vi "UHR-Fleezers Control (host) - 12.5.vi"() -> ()   [LabVIEW 2012] (continued)
            "Threshold stored (nm)" <- w2740
          }
        }
      }
      event "FB Trig Integrate": Value Change {
        n1853 = event-data() -> ()  [unwired: 7 out]
        n1854 = local read "FB Trig Integrate"() -> (w2742:u32)
        n1855 = xnode "Read/Write Control"("FPGA VI Reference In"=w2744, "error in"=w2743, "FB Trig Integrate"=w2742) -> ("error out"=w2741:errorcluster)  [unwired: 1 out]
      }
      event "11": Value Change {
        n1856 = event-data() -> ()  [unwired: 7 out]
        n1857 = local read "11"() -> (w2745:bool)
        n1858 = case shown="True" w2745 {
          frame False {
          }
          frame True {
            n1859 = local read "Messages"() -> (w2747:string)
            n1860 = call "Update messages.vi"("Message to add"="You kicked it up to 11!", "Old message string"=w2747) -> ("New message string"=w2748:string)
            n1861 = call <vilib>:"Beep.vi"() -> ()  [unwired: 12 in]
            n1862 = local write "Messages"(w2748) -> ()
          }
        }
      }
      event "Trap Pos. FB ON": Value Change {
        n1863 = event-data() -> ()  [unwired: 7 out]
        n1864 = xnode "Read/Write Control"("FPGA VI Reference In"=w2751, "error in"=w2750, "Force feedback"="Trap Pos. FB ON") -> ()  [unwired: 2 out]
      }
      event "Remove Action Offset": Value Change {
        n1865 = event-data() -> ()  [unwired: 7 out]
        n1866 = local write "Remove Action Offset"(FALSE ("Remove Action Offset")) -> ()
        n1867 = local read "Trap Pos. FB Mult Factor"() -> (w2756:i64)
        n1868 = local read "Trap Pos FB Action"() -> (w2754:i64)
        n1869 = local read "Trap Pos. FB Offset Factor"() -> (w2752:i64)
        n1870 = Multiply(x=w2756, y=w2754) -> (x*y=w2755:i64)
        n1871 = Add(x=w2755, y=w2752) -> (x+y=w2753:i64)
        n1872 = local write "Trap Pos. FB Offset Factor"(w2753) -> ()
        n1873 = xnode "Read/Write Control"("FPGA VI Reference In"=w2759, "error in"=w2758, "Trap Pos. FB Offset Factor"=w2753) -> ()  [unwired: 2 out]
      }
      event "Remove Unwinding Offset": Value Change {
        n1874 = event-data() -> ()  [unwired: 7 out]
        n1875 = local write "Remove Unwinding Offset"(FALSE ("Remove Action Offset")) -> ()
        n1876 = local read "Trap Pos. FB Mult Factor"() -> (w2771:i64)
        n1877 = local read "Trap Pos FB Action"() -> (w2769:i64)
        n1878 = local read "Trap Pos. FB Offset Factor"() -> (w2768:i64)
        n1879 = Multiply(x=w2771, y=w2769) -> (x*y=w2770:i64)
        n1880 = local read "Trap Pos. FB Mult Factor"() -> (w2767:i64)
        n1881 = Add(x=w2770, y=w2768) -> (x+y=w2761:i64)
        n1882 = Multiply(x=32768, y="factor") -> (x*y=w2764:dbl)
        n1883 = Multiply(x=w2764, y=w2767) -> (x*y=w2766:dbl)
        n1884 = Subtract(x=w2761, y=w2766) -> (x-y=w2765:dbl)
        n1885 = To Quad Integer(1:w2765) -> (0:w2760:i64)
        n1886 = xnode "Read/Write Control"("FPGA VI Reference In"=w2774, "error in"=w2773, "Trap Pos. FB Offset Factor"=w2760) -> ()  [unwired: 2 out]
        n1887 = local write "Trap Pos. FB Offset Factor"(w2760) -> ()
      }
      event "Trap Pos. FB Range", "Trap Pos. FB Gains", "Trap Pos. FB Mult Factor", "Trap Pos. FB Offset Factor", "Trap Pos FB Negate Action", "Trap Pos FB Monitor\nT1 or T2", "Differential FB?", "Negate Diff?": Value Change {
        n1888 = event-data() -> ()  [unwired: 7 out]
        n1889 = Unbundle By Name("Trap Pos. FB Gains") -> ("proportional gain (Kc)"=w2777:fxp<+/-,16,8>, "integral gain (Kc*Ts/Ti)"=w2776:fxp<+/-,16,8>, "derivative gain (Kc*Td/Ts)"=w2775:fxp<+/-,16,8>)
        n1890 = local read "Negate Diff?"() -> (w2782:bool)
        n1891 = Unbundle By Name("Trap Pos. FB Range") -> ("output high"=w2780:fxp<+/-,16,1>, "output low"=w2779:fxp<+/-,16,1>)
        n1892 = xnode "Read/Write Control"("FPGA VI Reference In"=w2790, "error in"=w2789, "FB2 output high"=w2780, "FB2 output low"=w2779, "P2"=w2777, "I2"=w2776, "D2"=w2775, "Trap Pos. FB Mult Factor"="Trap Pos. FB Mult Factor", "Trap Pos. FB Offset Factor"="Trap Pos. FB Offset Factor", "Trap Pos FB Negate Action"="Trap Pos FB Negate Action", "Trap Pos FB Monitor T1 or T2"="Trap Pos FB Monitor\nT1 or T2", "AI1 X Scale"="Trap Pos. AI1 X Pre-scale", "Negate Diff?"=w2782, "Diff FB Measurement?"="Differential FB?") -> ()  [unwired: 2 out]
      }
      event "Trap Pos FB SP", "Trap Pos FB SP 2", "Use SP 2": Value Change {
        n1893 = event-data() -> ()  [unwired: 7 out]
        n1894 = Select(t="Trap Pos FB SP 2", s="Use SP 2", f="Trap Pos FB SP") -> (s? t:f=w2791:fxp<+/-,16,1>)
        n1895 = xnode "Read/Write Control"("FPGA VI Reference In"=w2796, "error in"=w2795, "Trap Pos. FB SP"=w2791) -> ()  [unwired: 2 out]
      }
      event "Offset SP2 from SP1": Value Change {
        n1896 = event-data() -> ()  [unwired: 7 out]
        n1897 = local read "Trap Pos FB SP"() -> (w2799:fxp<+/-,16,1>)
        n1898 = Add(x=w2799, y="SP2 Offset") -> (x+y=w2797:fxp<+/-,16,1>)
        n1899 = property on="Trap Pos FB SP 2" class="DigNum (strict)"("Val(Sgnl)"=w2797) -> ()  [unwired: 2 in, 2 out]
        n1900 = local write "Offset SP2 from SP1"(FALSE ("Offset SP2 from SP1")) -> ()
      }
      event "Set Reading to\nSetpoint": Value Change {
        # "This is the actual PID input signal"
        n1901 = event-data() -> ()  [unwired: 7 out]
        n1902 = local write "Set Reading to\nSetpoint"(FALSE ("Set SP to Reading")) -> ()
        n1903 = xnode "Read/Write Control"("FPGA VI Reference In"=w2805, "error in"=w2804) -> ("FPGA VI Reference Out"=w2803:T20, "error out"=w2802:errorcluster, "Trap Pos FB Int-Norm Signal"=w2801:fxp<+/-,16,1>)
        n1904 = local read "Differential FB?"() -> (w2806:bool)
        n1905 = case shown="False" w2806 {
          tunnel: [w2811 w2818] -> w2808
          tunnel: w2801 -> [w2809 w2818]
          frame False {
            n1906 = local read "Trap Pos FB Monitor\nT1 or T2"() -> (w2814:bool)
            n1907 = local read "Trap X AI1 (DMA)"() -> (w2817:T13)
            n1908 = Unbundle By Name(w2817) -> ("Set 1"=w2816:fxp<+/-,16,1>, "Set 2"=w2815:fxp<+/-,16,1>)
            n1909 = Select(t=w2816, s=w2814, f=w2815) -> (s? t:f=w2813:fxp<+/-,16,1>)
            n1910 = Not(x="Set SP Using...") -> (.not. x?=w2810:bool)
            n1911 = Select(t=w2809, s=w2810, f=w2813) -> (s? t:f=w2811:fxp<+/-,16,1>)
          }
          frame True {
          }
        }
        n1912 = xnode "Read/Write Control"("FPGA VI Reference In"=w2803, "error in"=w2802, "Trap Pos. FB SP"=w2808) -> ()  [unwired: 2 out]
        n1913 = local write "Trap Pos FB SP"(w2808) -> ()
      }
      event "Trap Pos. FB Out Scale 2^n": Value Change {
        n1914 = event-data() -> ()  [unwired: 7 out]
        n1915 = Scale By Power Of 2(n="Trap Pos. FB Out Scale 2^n", x=ext 1.0) -> (x*2^n=w2819:ext)
        n1916 = property on="Trap Pos. FB Mult Factor" class="DigNum (strict)"("Val(Sgnl)"=w2819) -> ()  [unwired: 2 in, 2 out]
      }
      event "Trap Pos FB Int Count": Value Change {
        n1917 = event-data() -> ()  [unwired: 7 out]
        n1918 = xnode "Read/Write Control"("FPGA VI Reference In"=w2824, "error in"=w2823, "Trap Pos FB Int Count"="Trap Pos FB Int Count") -> ()  [unwired: 2 out]
      }
      event "Trap pos": Value Change {
        n1919 = event-data() -> ()  [unwired: 7 out]
        n1920 = case shown="True" "Trap pos" {
          frame False {
            n1921 = property on="Trap Delta Graph" class="WFGraph (strict)"("Visible"=TRUE) -> ()  [unwired: 2 in, 2 out]
            n1922 = property on="Saved trap pos" class="WFGraph (strict)"("Visible"=FALSE) -> ()  [unwired: 2 in, 2 out]
          }
          frame True {
            n1923 = property on="Saved trap pos" class="WFGraph (strict)"("Visible"=TRUE) -> ()  [unwired: 2 in, 2 out]
            n1924 = property on="Trap Delta Graph" class="WFGraph (strict)"("Visible"=FALSE) -> ()  [unwired: 2 in, 2 out]
          }
        }
      }
    }
    "error out 2" <- w1634
    n1925 = node-c288() -> ()  [unwired: 2 out]
  }
  n1926 = while "Duncan's play event loop" {
    stop <- w2831 stop-if-true
    n1927 = Create User Event(user event datatype=TRUE ("Boolean")) -> (user event=w2832:refnum<user-event>)  [unwired: 1 in, 1 out]
    n1928 = Create User Event(user event datatype=TRUE ("Boolean")) -> (user event=w2839:refnum<user-event>)  [unwired: 1 in, 1 out]
    n1929 = global write "Global for fluorescence simulation mean (30 samples), (power series).vi" "Red Signal"(w2832) -> ()
    n1930 = global write "Global for fluorescence simulation mean (30 samples), (power series).vi" "Green Signal"(w2839) -> ()
    n1931 = register-events(w2839, w2832) -> (reference out=w2838:refnum<event-registration>)  [unwired: 2 in, 1 out]
    n1932 = event shown="[1] \"Get Fluorophore\": Value Change" {
      selector: w2838 -> [_ _ _ _]
      dyn-events: _ -> [_ _ _ _]
      timeout: 100 -> [_ _ _ _]
      event Timeout {
        n1933 = event-data() -> ()  [unwired: 1 in, 2 out]
      }
      event "Get Fluorophore": Value Change {
        n1934 = event-data() -> ("OldVal"=w2841:bool)  [unwired: 1 in, 4 out]
        n1935 = case shown="True" w2841 {
          selector: w2841 -> [_ w2842]
          frame False {
          }
          frame True {
            n1936 = property on="Move to Position 3" class="Bool"("Val(Sgnl)"=w2842) -> ()  [unwired: 2 in, 2 out]
            n1937 = case shown="1" "Numeric" {
              frame 0, Default {
              }
              frame 1 {
                n1938 = property on="Green Laser ON" class="Bool (strict)"("Val(Sgnl)"=TRUE ("Value (Signaling)")) -> ()  [unwired: 2 in, 2 out]
              }
              frame 2 {
                n1939 = property on="Red Laser ON" class="Bool (strict)"("Val(Sgnl)"=TRUE) -> ()  [unwired: 2 in, 2 out]
              }
            }
          }
        }
      }
      event User Event {
        n1940 = event-data() -> ("Boolean"=w2846:bool)  [unwired: 1 in, 3 out]
        "Green Fluorophore" <- w2846
        n1941 = property on="Get Fluorophore" class="Bool (strict)"("Val(Sgnl)"=w2846) -> ()  [unwired: 2 in, 2 out]
      }
      event User Event {
        n1942 = event-data() -> ("Boolean"=w2847:bool)  [unwired: 1 in, 3 out]
        "Red Fluorophore" <- w2847
        n1943 = property on="Get Fluorophore" class="Bool (strict)"("Val(Sgnl)"=w2847) -> ()  [unwired: 2 in, 2 out]
      }
    }
    n1944 = property on="Get Fluorophore" class="Bool (strict)"("Val(Sgnl)"="Get Fluorophore") -> ()  [unwired: 2 in, 2 out]
    n1945 = Wait (ms)(milliseconds to wait=u32 100) -> ()  [unwired: 1 out]
    n1946 = local read "Stop All"() -> (w2830:bool)
    n1947 = Or(x=w2830, y="stop") -> (x .or. y?=w2831:bool)
  }
  n1948 = timed-loop "Mouse control: trap position (AOM deflection), set confocal spot from image" {
    tunnel: [w2849] -> w207
    tunnel: w13 -> [w2848]
    timing: w129 -> [_]
    timing-out: [_] -> w128
    stop <- w2849 stop-if-true
    n1949 = node-c288() -> ()  [unwired: 2 out]
    n1950 = event shown="[0] \"Pane\": Mouse Down" {
      selector: _ -> [_ _]
      dyn-events: _ -> [_ _]
      timeout: _ -> [_ _]
      tunnel: w2848 -> [w2852 _]
      event Mouse Down {
        n1951 = event-data() -> ("Time"=w2854:u32, "Coords"=w2853:T7, "Button"=w2855:u16)  [unwired: 6 out]
        n1952 = case shown="1" w2855 {
          tunnel: w2854 -> [_ _ w2961]
          tunnel: w2853 -> [_ w2892 w2959]
          tunnel: w2852 -> [_ _ w2957]
          frame 0, Default {
          }
          frame 1 {
            n1953 = property on="APD 2" class="ImageControl"() -> ("Displayed Image Position"=w2862:cluster{"Left":i32, "Top":i32})  [unwired: 2 in, 2 out]
            n1954 = property on="APD 1" class="ImageControl"() -> ("Displayed Image Position"=w2891:cluster{"Left":i32, "Top":i32})  [unwired: 2 in, 2 out]
            n1955 = property on="Detection Laser X" class="ImageControl"() -> ("Displayed Image Position"=w2888:cluster{"Left":i32, "Top":i32})  [unwired: 2 in, 2 out]
            n1956 = property on="Detection Laser Y" class="ImageControl"() -> ("Displayed Image Position"=w2887:cluster{"Left":i32, "Top":i32})  [unwired: 2 in, 2 out]
            n1957 = property on="APD 2" class="ImageControl"() -> ("Displayed Image Size"=w2861:cluster{"Width":u32, "Height":u32})  [unwired: 2 in, 2 out]
            n1958 = property on="APD 1" class="ImageControl"() -> ("Displayed Image Size"=w2889:cluster{"Width":u32, "Height":u32})  [unwired: 2 in, 2 out]
            n1959 = property on="Detection Laser X" class="ImageControl"() -> ("Displayed Image Size"=w2890:cluster{"Width":u32, "Height":u32})  [unwired: 2 in, 2 out]
            n1960 = property on="Detection Laser Y" class="ImageControl"() -> ("Displayed Image Size"=w2886:cluster{"Width":u32, "Height":u32})  [unwired: 2 in, 2 out]
            n1961 = Unbundle By Name(w2861) -> ("Width"=w2858:u32, "Height"=w2857:u32)
            n1962 = Unbundle By Name(w2862) -> ("Left"=w2860:i32, "Top"=w2859:i32)
            n1963 = Unbundle By Name(w2889) -> ("Width"=w2883:u32, "Height"=w2882:u32)
            n1964 = Unbundle By Name(w2890) -> ("Width"=w2879:u32, "Height"=w2878:u32)
            n1965 = Unbundle By Name(w2886) -> ("Width"=w2875:u32, "Height"=w2874:u32)
            n1966 = Unbundle By Name(w2891) -> ("Left"=w2885:i32, "Top"=w2884:i32)
            n1967 = Unbundle By Name(w2888) -> ("Left"=w2881:i32, "Top"=w2880:i32)
            n1968 = Unbundle By Name(w2887) -> ("Left"=w2877:i32, "Top"=w2876:i32)
            n1969 = Bundle("Left"=w2860, "Top"=w2859, "Width"=w2858, "Height"=w2857) -> (w2856:T32)  [unwired: 1 in]
            n1970 = Bundle("Left"=w2885, "Top"=w2884, "Width"=w2883, "Height"=w2882) -> (w2873:T32)  [unwired: 1 in]
            n1971 = Bundle("Left"=w2881, "Top"=w2880, "Width"=w2879, "Height"=w2878) -> (w2872:T32)  [unwired: 1 in]
            n1972 = Bundle("Left"=w2877, "Top"=w2876, "Width"=w2875, "Height"=w2874) -> (w2871:T32)  [unwired: 1 in]
            n1973 = Build Cluster Array(w2856, w2873, w2872, w2871) -> (w2870:T33)
            n1974 = for {
              tunnel: w2892 -> [w2903]
              tunnel: w2870 -> [w2904] mode=indexing
              shift-right: [w2901] -> w2868
              shift-left: TRUE -> [w2902]
              shift-right: [w2900] -> w2866
              shift-left: _ -> [w2896]
              shift-right: [w2899] -> w2865
              shift-left: _ -> [w2895]
              shift-right: [w2898] -> w2864
              shift-left: _ -> [w2894]
              shift-right: [w2897] -> w2863
              shift-left: _ -> [w2893]
              n1975 = case shown="True" w2902 {
                selector: w2902 -> [w2909 _]
                tunnel: w2904 -> [_ w2918]
                tunnel: w2903 -> [_ w2916]
                tunnel: [w2909 w2914] -> w2901
                tunnel: [w2908 w2913] -> w2900
                tunnel: [w2907 w2912] -> w2899
                tunnel: [w2906 w2911] -> w2898
                tunnel: [w2905 w2910] -> w2897
                tunnel: w2896 -> [w2908 _]
                tunnel: w2895 -> [w2907 _]
                tunnel: w2894 -> [w2906 _]
                tunnel: w2893 -> [w2905 _]
                frame False {
                }
                frame True {
                  n1976 = Unbundle(w2918) -> (w2917:T32)
                  n1977 = call "isclickinwindow.vi"("Image Param"=w2917, "Point32"=w2916) -> ("4 Y"=w2910:i32, "3 Height"=w2911:i32, "2 X"=w2912:i32, "1 Width"=w2913:i32, "In image?"=w2915:bool)  [unwired: 1 in]
                  n1978 = Not(x=w2915) -> (.not. x?=w2914:bool)
                }
              }
            }
            n1979 = Not(x=w2868) -> (.not. x?=w2867:bool)
            n1980 = case shown="True" w2867 {
              tunnel: w2865 -> [_ w2932]
              tunnel: w2863 -> [_ w2931]
              tunnel: w2866 -> [_ w2930]
              tunnel: w2864 -> [_ w2929]
              frame False {
              }
              frame True {
                w2919 = FALSE ("Get Point")
                n1981 = local read "Scan lines (y)"() -> (w2934:u64)
                n1982 = disable-structure shown="Disabled" {
                  frame Disabled {
                  }
                  frame Enabled {
                  }
                }
                n1983 = local read "Actual MCL Inc (V)"() -> (w2928:dbl)
                n1984 = local read "Scan steps (MCL)"() -> (w2933:u64)
                n1985 = Divide "Y Pix/step"(x=w2929, y=w2934) -> (x/y=w2941:dbl)
                n1986 = Divide "Y V/pix"(x=w2928, y=w2941) -> (x/y=w2940:dbl)
                n1987 = Divide "Y half step offset"(x=w2928, y=2.0) -> (x/y=w2942:dbl)
                n1988 = Divide "X pix/step"(x=w2930, y=w2933) -> (x/y=w2939:dbl)
                n1989 = Negate(x=w2942) -> (-x=w2943:dbl)
                n1990 = local read "Initial Y"() -> (w2949:dbl)
                n1991 = Multiply(x=w2931, y=w2940) -> (x*y=w2950:dbl)
                n1992 = Divide "X half step offset"(x=w2928, y=2.0) -> (x/y=w2936:dbl)
                n1993 = Divide "X V/pix"(x=w2928, y=w2939) -> (x/y=w2938:dbl)
                n1994 = Multiply(x=w2928, y=w2933) -> (x*y=w2945:dbl)
                n1995 = Compound Arithmetic op=ADD(w2943, w2950, w2949) -> (w2920:dbl)
                "Pointer Y (V)" <- w2920
                n1996 = Multiply(x=w2938, y=w2932) -> (x*y=w2947:dbl)
                n1997 = Negate(x=w2936) -> (-x=w2935:dbl)
                n1998 = local read "Initial X"() -> (w2948:dbl)
                n1999 = Negate(x=w2947) -> (-x=w2946:dbl)
                n2000 = Compound Arithmetic op=ADD(w2935, w2945, w2948, w2946) -> (w2921:dbl)
                "Pointer X (V)" <- w2921
                n2001 = case shown="True" "Set High F Confocal Spot (X-Y)" {
                  tunnel: w2921 -> [_ w2951]
                  tunnel: w2920 -> [_ w2952]
                  frame False {
                  }
                  frame True {
                    "Confocal Y 2 (V)" <- w2952
                    "Confocal X 2 (V)" <- w2951
                  }
                }
                n2002 = Or(x="Set X Only", y="Set Confocal Spot (X-Y)") -> (x .or. y?=w2924:bool)
                n2003 = Or(x="Set Confocal Spot (X-Y)", y="Set Y Only") -> (x .or. y?=w2923:bool)
                n2004 = case shown="True" w2924 {
                  tunnel: w2921 -> [_ w2953]
                  frame False {
                  }
                  frame True {
                    n2005 = property on="AO2" class="Slide (strict)"("Val(Sgnl)"=w2953) -> ()  [unwired: 2 in, 2 out]
                    "Confocal X 1 (V)" <- w2953
                  }
                }
                n2006 = case shown="True" w2923 {
                  tunnel: w2920 -> [_ w2954]
                  frame False {
                  }
                  frame True {
                    n2007 = property on="AO1" class="Slide (strict)"("Val(Sgnl)"=w2954) -> ()  [unwired: 2 in, 2 out]
                    "Confocal Y 1 (V)" <- w2954
                  }
                }
                n2008 = local write "Set High F Confocal Spot (X-Y)"(w2919) -> ()
                n2009 = local write "Set Confocal Spot (X-Y)"(w2919) -> ()
                n2010 = local write "Set X Only"(w2919) -> ()
                n2011 = local write "Set Y Only"(w2919) -> ()
              }
            }
          }
          frame 3 {
            n2012 = local read "BD 2 Frequency 1 (MHz)"() -> (w2955:dbl)
            n2013 = local read "BD 1 Frequency 1 (MHz)"() -> (w2956:dbl)
            n2014 = local write "Manipulating Trap"(TRUE ("Manipulating Trap")) -> ()
            n2015 = local write "Coords"(T7 {"Horizontal"=0, "Vertical"=0} ("Coords")) -> ()
            n2016 = while {
              tunnel: w2961 -> [w2966]
              tunnel: w2959 -> [w2965]
              tunnel: w2957 -> [w2964]
              tunnel: w2956 -> [w2963]
              tunnel: w2955 -> [w2962]
              stop <- w2967 stop-if-true
              n2017 = event shown="[0] \"Pane\": Mouse Move" {
                selector: _ -> [_ _]
                dyn-events: _ -> [_ _]
                timeout: _ -> [_ _]
                tunnel: ["Force Manip Abort" w3031] -> w2967
                tunnel: w2966 -> [w2974 _]
                tunnel: w2965 -> [w2972 _]
                tunnel: w2964 -> [w2971 _]
                tunnel: w2963 -> [w2970 _]
                tunnel: w2962 -> [w2969 _]
                event Mouse Move {
                  n2018 = event-data() -> ("Time"=w2975:u32, "Coords"=w2976:T7)  [unwired: 3 out]
                  n2019 = Less?(x=w2975, y=w2974) -> (x < y?=w2973:bool)
                  n2020 = case "Makes sure old motion events prior to mouse click aren't used" shown="False" w2973 {
                    tunnel: w2976 -> [w3018 _]
                    tunnel: w2972 -> [w3019 _]
                    tunnel: w2971 -> [w2996 _]
                    tunnel: w2970 -> [w2992 _]
                    tunnel: w2969 -> [w2991 _]
                    frame False {
                      n2021 = Subtract(x=w3018, y=w3019) -> (x-y=w3017:T7)
                      "Coords" <- w3017
                      n2022 = local read "Y RF Frequency Limits (MHz)"() -> (w2977:T16)
                      n2023 = To Double Precision Float(number=w3017) -> (double precision float=w3016:cluster{"Horizontal":dbl, "Vertical":dbl})
                      n2024 = Multiply(x=cluster{"Horizontal":dbl, "Vertical":dbl} {"Horizontal"=-1.0, "Vertical"=1.0}, y="Manipulation Scaling") -> (x*y=w3012:cluster{"Horizontal":dbl, "Vertical":dbl})
                      n2025 = local read "X RF Frequency Limits (MHz)"() -> (w2978:T16)
                      n2026 = Multiply(x=w3016, y=w3012) -> (x*y=w3014:cluster{"Horizontal":dbl, "Vertical":dbl})
                      n2027 = Unbundle By Name(w3014) -> ("Horizontal"=w3009:dbl, "Vertical"=w3013:dbl)
                      n2028 = Unbundle By Name(w2977) -> ("Maximum"=w2980:dbl, "Minimum"=w2979:dbl)
                      n2029 = Boolean To (0,1)(Boolean="Manip. X?") -> (0, 1=w3007:i16)
                      n2030 = Boolean To (0,1)(Boolean="Manip. Y?") -> (0, 1=w3004:i16)
                      n2031 = local read "BD 1 Frequency 2 (MHz)"() -> (w2994:dbl)
                      n2032 = Multiply(x=w3013, y=w3004) -> (x*y=w3006:dbl)
                      n2033 = Multiply(x=w3007, y=w3009) -> (x*y=w3010:dbl)
                      n2034 = local read "BD 2 Frequency 2 (MHz)"() -> (w2993:dbl)
                      n2035 = Unbundle By Name(w2978) -> ("Maximum"=w2982:dbl, "Minimum"=w2981:dbl)
                      n2036 = Add(x=w2991, y=w3006) -> (x+y=w2984:dbl)
                      n2037 = Add(x=w2992, y=w3010) -> (x+y=w2986:dbl)
                      n2038 = In Range and Coerce(upper limit=w2982, x=w2986, lower limit=w2981) -> (coerced(x)=w2985:dbl)  [unwired: 1 out]
                      n2039 = In Range and Coerce(upper limit=w2980, x=w2984, lower limit=w2979) -> (coerced(x)=w2983:dbl)  [unwired: 1 out]
                      n2040 = Subtract(x=w2985, y=w2994) -> (x-y=w3003:dbl)
                      n2041 = Subtract(x=w2983, y=w2993) -> (x-y=w3002:dbl)
                      n2042 = Square(x=w3003) -> (x^2=w3001:dbl)
                      n2043 = Square(x=w3002) -> (x^2=w3000:dbl)
                      n2044 = Add(x=w3001, y=w3000) -> (x+y=w2999:dbl)
                      n2045 = Square Root(x=w2999) -> (sqrt(x)=w2995:dbl)
                      n2046 = In Range and Coerce(upper limit="Limit Max (MHz)", x=w2995, lower limit="Limit Min (MHz)") -> (In Range?=w2988:bool)  [unwired: 1 out]
                      n2047 = Not(x="Limits Enable") -> (.not. x?=w2987:bool)
                      n2048 = Or(x=w2988, y=w2987) -> (x .or. y?=w2989:bool)
                      n2049 = case shown="True" w2989 {
                        tunnel: w2996 -> [_ w3029]
                        tunnel: w2995 -> [_ w3020]
                        tunnel: w2985 -> [_ w3027]
                        tunnel: w2994 -> [_ w3026]
                        tunnel: w2983 -> [_ w3025]
                        tunnel: w2993 -> [_ w3024]
                        tunnel: w2978 -> [_ w3022]
                        tunnel: w2977 -> [_ w3021]
                        frame False {
                        }
                        frame True {
                          n2050 = local read "BD 1 Frequency 3 (MHz)"() -> (w3028:dbl)
                          n2051 = local read "BD 2 Frequency 3 (MHz)"() -> (w3023:dbl)
                          n2052 = local write "Trap Delta (MHz)"(w3020) -> ()
                          n2053 = call "set RF board frequency - interlace.vi"("Board 2 Frequency Limits"=w3021, "Board 1 Frequency Limits"=w3022, "FPGA VI Reference In"=w3029, "Board 2 Frequency 3 (MHz)"=w3023, "Board 1 Frequency 3 (MHz)"=w3028, "Board 2 Frequency 2 (MHz)"=w3024, "Board 2 Frequency 1 (MHz)"=w3025, "Board 1 Frequency 2 (MHz)"=w3026, "Board 1 Frequency 1  (MHz)"=w3027) -> ()  [unwired: 1 in, 2 out]
                          n2054 = local write "BD 2 Frequency 1 (MHz)"(w3025) -> ()
                          n2055 = local write "BD 1 Frequency 1 (MHz)"(w3027) -> ()
                        }
                      }
                    }
                    frame True {
                    }
                  }
                }
                event Mouse Up {
                  n2056 = event-data() -> ("Button"=w3030:u16)  [unwired: 8 out]
                  n2057 = case shown="3" w3030 {
                    tunnel: [FALSE TRUE] -> w3031
                    frame 0, Default {
                    }
                    frame 3 {
                      n2058 = local read "Trap Delta (MHz)"() -> (w3033:dbl)
                      n2059 = property on="Initial delta (MHz)" class="DigNum (strict)"("Val(Sgnl)"=w3033) -> ()  [unwired: 2 in, 2 out]
                      n2060 = local write "Manipulating Trap"(FALSE ("Manipulating Trap")) -> ()
                    }
                  }
                }
              }
            }
          }
        }
      }
      event Mouse Move {
        n2061 = event-data() -> ()  [unwired: 6 out]
      }
    }
    n2062 = local read "Stop All"() -> (w2849:bool)
    n2063 = node-c288() -> ()  [unwired: 2 out]
  }
  n2064 = timed-loop "Main data acquisition loop (get data, process data for display, and save data to disk)" {
    tunnel: w12 -> [w3345]
    tunnel: w88 -> [w3344]
    tunnel: [w3374] -> w292
    tunnel: [w3369] -> w290
    timing: w200 -> [_]
    timing-out: [_] -> w199
    tunnel: w105 -> [w3198]
    stop <- "Stop All" stop-if-true
    w3115 = "Initialize"
    # "Fluorescence data into FIFO for external control vi's\n(e.g., fluorescence triggering) - Duncan Nall"
    n2065 = node-c288() -> ()  [unwired: 2 out]
    n2066 = First Call?() -> (First Call?: T/F=w3150:bool)
    n2067 = Or(x="Reset", y=w3150) -> (x .or. y?=w3151:bool)
    n2068 = local read "Flushing P1"() -> (w3070:bool)
    n2069 = case "Reset data stream (manual reset or at begining of some rastering and imaging)" shown="True" w3151 {
      tunnel: w3345 -> [w4421 w4429]
      tunnel: w3344 -> [w4420 w4428]
      tunnel: [w4421 w4423] -> w3340
      tunnel: [w4420 w4422] -> w3339
      frame False {
      }
      frame True {
        w4426 = TRUE ("AI to FIFO")
        n2070 = local write "Overflow (data lost)"(FALSE ("Overflow (data lost)")) -> ()
        n2071 = call "reset FPGA DMA.vi"("error in"=w4428, "FPGA VI Reference In"=w4429) -> ("error out"=w4424:errorcluster, "FPGA VI Reference Out"=w4425:T20)
        n2072 = xnode "Read/Write Control"("FPGA VI Reference In"=w4425, "error in"=w4424, "AI to FIFO"=w4426, "APD to FIFO"=w4426) -> ("FPGA VI Reference Out"=w4423:T20, "error out"=w4422:errorcluster)
      }
    }
    n2073 = case shown="True" w3070 {
      frame False {
      }
      frame True {
        n2074 = local read "Flush rate (uL/m) P1"() -> (w3404:dbl)
        n2075 = local read "HP1 Flush Time (s)"() -> (w3413:dbl)
        n2076 = local read "DMA Update Period (s)"() -> (w3407:dbl)
        n2077 = Divide(x=w3404, y=60.0) -> (x/y=w3405:dbl)
        n2078 = Divide(x=w3413, y=w3407) -> (x/y=w3402:dbl)
        n2079 = feedback #1(0) -> (w3411:i32)
        n2080 = Increment(x=w3411) -> (x+1=w3401:i32)
        n2081 = Greater?(x=w3401, y=w3402) -> (0:w3410:bool)
        n2082 = Compound Arithmetic op=MULTIPLY(w3407, w3401, w3405) -> (→"P1 Flush Volume (uL)":dbl)
        n2083 = Divide(x=w3401, y=w3402) -> (x/y=→"P1 Flushing Bar":dbl)
        n2084 = case shown="True" w3410 {
          tunnel: w3401 -> [w3414 _]
          tunnel: [w3414 0] -> w3409
          frame False {
          }
          frame True {
            w3415 = FALSE ("Flushing P1")
            n2085 = local write "Inject Pump 1"(w3415) -> ()
            n2086 = local write "Flushing P1"(w3415) -> ()
            n2087 = property on="Clear Volume P1" class="Bool (strict)"("Val(Sgnl)"=TRUE ("Value (Signaling)")) -> ()  [unwired: 2 in, 2 out]
          }
        }
        n2088 = feedback-in #1(w3409) -> ()
      }
    }
    n2089 = Or(x="Start AOD Scan", y="Trap Raster Scan") -> (x .or. y?=w3296:bool)
    n2090 = case "Start AOM raster scan" shown="True" w3296 {
      tunnel: w3340 -> [w4271 w4281]
      tunnel: w3339 -> [w4270 w4280]
      tunnel: [w4271 w4274] -> w3338
      tunnel: [w4270 w4273] -> w3337
      frame False {
      }
      frame True {
        n2091 = case shown="True" "Restart DMA? (AOD)" {
          tunnel: [w4319 w4321] -> w4275
          tunnel: [w4318 w4320] -> w4276
          tunnel: w4281 -> [w4319 w4323]
          tunnel: w4280 -> [w4318 w4322]
          frame False {
          }
          frame True {
            n2092 = local write "Overflow (data lost)"(FALSE ("Overflow (data lost)")) -> ()
            n2093 = call "reset FPGA DMA.vi"("error in"=w4322, "FPGA VI Reference In"=w4323) -> ("error out"=w4320:errorcluster, "FPGA VI Reference Out"=w4321:T20)
          }
        }
        n2094 = local write "Trap Raster Scan"(FALSE ("Trap Raster Scan")) -> ()
        n2095 = case shown="True" "Move MCL Also?" {
          tunnel: w4276 -> [w4284 w4313]
          tunnel: w4275 -> [w4285 w4314]
          tunnel: [w4283 w4317] -> w4274
          tunnel: [w4282 w4316] -> w4273
          frame False {
            w4286 = TRUE ("AI to FIFO")
            n2096 = xnode "Read/Write Control"("FPGA VI Reference In"=w4285, "error in"=w4284, "AI to FIFO"=w4286, "APD to FIFO"=w4286, "Start scan"=w4286) -> ("FPGA VI Reference Out"=w4283:T20, "error out"=w4282:errorcluster)
          }
          frame True {
            w4310 = FALSE ("1D or 2D Scan?")
            w4315 = TRUE ("AI to FIFO")
            # "Count for MCL loop"
            # "N total cycles"
            # "N steps"
            # "V_int"
            n2097 = local read "Scan Range (nm)"() -> (w4292:dbl)
            n2098 = local read "Number of F/B Scans (AOD)"() -> (w4309:u16)
            n2099 = Sign(1:w4292) -> (0:w4291:dbl)
            n2100 = Compound Arithmetic op=MULTIPLY(w4292, "MCL Step Position Ratio", "MCL/AOM Scale Tweak") -> (w4296:dbl)
            n2101 = Negate(x=w4291) -> (-x=w4288:dbl)
            n2102 = Multiply(x=w4288, y="MCL Step Increment (V_int)") -> (x*y=w4290:dbl)
            n2103 = Divide(x=w4296, y="MCL X Cal (nm/V)") -> (x/y=w4302:dbl)
            n2104 = Multiply(x=32767.0 ("y"), y=w4302) -> (x*y=w4308:dbl)
            n2105 = local read "Total Counts (ticks)"() -> (w4293:u16)
            n2106 = local read "Cycles/step (AOD)"() -> (w4304:u64)
            n2107 = local read "Scan steps (AOD)"() -> (w4305:u64)
            n2108 = Divide(x=w4308, y=10.0) -> (x/y=w4301:dbl)
            n2109 = Divide(x=w4301, y="MCL Step Increment (V_int)") -> (x/y=w4299:dbl)
            n2110 = Absolute Value(x=w4299) -> (abs(x)=w4287:dbl)
            n2111 = Compound Arithmetic op=MULTIPLY(w4305, w4304, w4293) -> (w4300:u64)
            n2112 = local write "wait to reset values"(w4315) -> ()
            n2113 = local write "MCL Scanning"(w4315) -> ()
            n2114 = Divide(x=w4300, y=w4287) -> (x/y=w4297:dbl)
            "MCL Count" <- w4297
            n2115 = xnode "Read/Write Control"("FPGA VI Reference In"=w4314, "error in"=w4313, "Scan steps (MCL)"=w4287, "Number of scans (MCL)"=w4309, "Cycles per step (MCL)"=u64 1, "Scan freq.  increment (MCL)"=w4290, "1D or 2D Scan?"=w4310, "MCL Scan Axis"=w4310, "Cont. Scan (MCL)"=w4310, "MCL count"=w4297) -> ("FPGA VI Reference Out"=w4312:T20, "error out"=w4311:errorcluster)
            n2116 = xnode "Read/Write Control"("FPGA VI Reference In"=w4312, "error in"=w4311, "AI to FIFO"=w4315, "APD to FIFO"=w4315, "Start scan"=w4315, "Start scan (MCL)"=w4315) -> ("FPGA VI Reference Out"=w4317:T20, "error out"=w4316:errorcluster)
          }
        }
        "Raster Scanning..." <- TRUE ("Scanning...")
      }
    }
    n2117 = local read "Flushing P3"() -> (w3071:bool)
    n2118 = case "Keep track of when Harvard Pump 3 is done flushing" shown="True" w3071 {
      frame False {
      }
      frame True {
        n2119 = local read "Flush rate (uL/m) P3"() -> (w3421:dbl)
        n2120 = local read "DMA Update Period (s)"() -> (w3423:dbl)
        n2121 = local read "HP3 Flush Time (s)"() -> (w3430:dbl)
        n2122 = Divide(x=w3421, y=60.0) -> (x/y=w3419:dbl)
        n2123 = feedback #2(0) -> (w3428:i32)
        n2124 = Increment(x=w3428) -> (x+1=w3422:i32)
        n2125 = Divide(x=w3430, y=w3423) -> (x/y=w3424:dbl)
        n2126 = Greater?(x=w3422, y=w3424) -> (0:w3427:bool)
        n2127 = Compound Arithmetic op=MULTIPLY(w3423, w3422, w3419) -> (→"P3 Flush Volume (uL)":dbl)
        n2128 = case shown="True" w3427 {
          tunnel: w3422 -> [w3431 _]
          tunnel: [w3431 0] -> w3426
          frame False {
          }
          frame True {
            w3432 = FALSE ("Flushing P3")
            n2129 = local write "Inject Pump 3"(w3432) -> ()
            n2130 = local write "Flushing P3"(w3432) -> ()
            n2131 = property on="Clear Volume P3" class="Bool (strict)"("Val(Sgnl)"=TRUE ("Value (Signaling)")) -> ()  [unwired: 2 in, 2 out]
          }
        }
        n2132 = feedback-in #2(w3426) -> ()
        n2133 = Divide(x=w3422, y=w3424) -> (x/y=→"P3 Flushing Bar":dbl)
      }
    }
    n2134 = And(x="Save scans", y=w3296) -> (x .and. y?=w3336:bool)
    n2135 = Compound Arithmetic op=OR("Start MCL Scan", "Confocal Image", "Confocal Linescan") -> (w3294:bool)
    n2136 = And(x="Save Data (MCL)", y=w3294) -> (x .and. y?=w3335:bool)
    n2137 = case "Start MCL raster scan" shown="True" w3294 {
      tunnel: w3338 -> [w3883 w3899]
      tunnel: w3337 -> [w3882 w3898]
      tunnel: [w3883 w3894] -> w3197
      tunnel: [w3882 w3893] -> w3196
      tunnel: [FALSE w3892] -> w3321
      tunnel: "Start MCL Scan" -> [_ w3887]
      tunnel: "Confocal Image" -> [_ w3886]
      tunnel: "Confocal Linescan" -> [_ _]
      frame False {
      }
      frame True {
        w3892 = TRUE
        n2138 = case shown="True" "Restart DMA? (MCL)" {
          tunnel: [w3944 w3946] -> w3897
          tunnel: [w3943 w3945] -> w3896
          tunnel: w3899 -> [w3944 w3949]
          tunnel: w3898 -> [w3943 w3948]
          frame False {
          }
          frame True {
            n2139 = call "reset FPGA DMA.vi"("error in"=w3948, "FPGA VI Reference In"=w3949) -> ("error out"=w3945:errorcluster, "FPGA VI Reference Out"=w3946:T20)
            n2140 = local write "Overflow (data lost)"(FALSE ("Overflow (data lost)")) -> ()
          }
        }
        n2141 = case shown="False" w3887 {
          selector: w3887 -> [_ w3903]
          tunnel: w3886 -> [w3902 _]
          tunnel: [w3902 w3903] -> w3885
          frame False {
            n2142 = property on="2D or 1D Scan" class="Bool (strict)"("Val(Sgnl)"=w3902) -> ()  [unwired: 2 in, 2 out]
            n2143 = property on="Confocal Image" class="Bool (strict)"("Value"=FALSE ("Start Confocal Map")) -> ()  [unwired: 2 in, 2 out]
          }
          frame True {
          }
        }
        n2144 = local write "MCL Scanning"(w3892) -> ()
        n2145 = local read "AO1"() -> (w3889:dbl)
        n2146 = local read "AO2"() -> (w3888:dbl)
        n2147 = case shown="True" "Center Scan" {
          tunnel: w3897 -> [w3910 w3942]
          tunnel: w3896 -> [w3909 w3941]
          tunnel: [w3908 w3940] -> w3894
          tunnel: [w3907 w3939] -> w3893
          tunnel: [w3905 w3926] -> w3891
          tunnel: [w3904 w3925] -> w3890
          tunnel: w3889 -> [w3905 w3931]
          tunnel: w3888 -> [w3904 w3934]
          tunnel: w3885 -> [_ _]
          frame False {
            w3906 = TRUE ("AI to FIFO")
            n2148 = xnode "Read/Write Control"("FPGA VI Reference In"=w3910, "error in"=w3909, "AI to FIFO"=w3906, "APD to FIFO"=w3906, "Start scan (MCL)"=w3906) -> ("FPGA VI Reference Out"=w3908:T20, "error out"=w3907:errorcluster)
          }
          frame True {
            w3938 = TRUE ("AI to FIFO")
            n2149 = local read "Scan steps (MCL)"() -> (w3917:u64)
            n2150 = local read "Scan lines (y)"() -> (w3913:u64)
            n2151 = local read "Fast Scan Dir"() -> (w3924:bool)
            n2152 = local read "Actual MCL Inc (V)"() -> (w3914:dbl)
            n2153 = Decrement(x=w3913) -> (x-1=w3912:u64)
            n2154 = Decrement(x=w3917) -> (x-1=w3916:u64)
            n2155 = Multiply(x=w3914, y=w3912) -> (x*y=w3911:dbl)
            n2156 = Divide(x=w3911, y=2.0) -> (x/y=w3921:dbl)
            n2157 = Multiply(x=w3914, y=w3916) -> (x*y=w3915:dbl)
            n2158 = Divide(x=w3915, y=2.0) -> (x/y=w3920:dbl)
            n2159 = Select(t=w3920, s=w3924, f=w3921) -> (s? t:f=w3919:dbl)
            n2160 = Select(t=w3921, s=w3924, f=w3920) -> (s? t:f=w3923:dbl)
            n2161 = Subtract(x=w3931, y=w3923) -> (x-y=w3922:dbl)
            n2162 = Subtract(x=w3934, y=w3919) -> (x-y=w3918:dbl)
            n2163 = local read "2D or 1D Scan"() -> (w3936:bool)
            n2164 = Not(x=w3924) -> (.not. x?=w3930:bool)
            n2165 = Not(x=w3936) -> (.not. x?=w3932:bool)
            n2166 = And(x=w3924, y=w3932) -> (x .and. y?=w3933:bool)
            n2167 = And(x=w3932, y=w3930) -> (x .and. y?=w3935:bool)
            n2168 = Select(t=w3934, s=w3935, f=w3918) -> (s? t:f=w3925:dbl)
            n2169 = Select(t=w3931, s=w3933, f=w3922) -> (s? t:f=w3926:dbl)
            n2170 = call "Volt to I16.vi"("Voltage In"=w3926) -> ("I16 Voltage Out"=w3929:i16)
            n2171 = call "Volt to I16.vi"("Voltage In"=w3925) -> ("I16 Voltage Out"=w3928:i16)
            n2172 = xnode "Read/Write Control"("FPGA VI Reference In"=w3942, "error in"=w3941, "AI to FIFO"=w3938, "APD to FIFO"=w3938, "Start scan (MCL)"=w3938, "AO1"=w3929, "AO2"=w3928) -> ("FPGA VI Reference Out"=w3940:T20, "error out"=w3939:errorcluster)
          }
        }
        "Initial Y" <- w3891
        "Initial X" <- w3890
        n2173 = local write "Tab Control 6"(T3."Imaging" ("Tab Control 6")) -> ()
        "wait to reset values" <- w3892
      }
    }
    n2174 = local read "APD Elements/DMA read"() -> (w3038:u32)
    n2175 = local read "Trap AI Elements/DMA read"() -> (w3259:u32)
    n2176 = xnode "Get APD Data"("FPGA VI Reference In"=w3197, "error in"=w3196, "Number of Elements"=w3038, "Timeout (ms)"=-1) -> ("Data"=w3228:u32[], "Elements Remaining"=→"APD FIFO Elements Remaining":u32)  [unwired: 2 out]
    n2177 = local read "Trap Pos Elements/DMA read"() -> (w3193:u32)
    n2178 = xnode "Invoke Method"("FPGA VI Reference In"=w3197, "error in"=w3196, "Number of Elements"=w3193, "Timeout (ms)"=-1) -> ("Data"=w3157:u16[], "Elements Remaining"=→"Trap Pos FIFO El Remaining":u32)  [unwired: 2 out]
    n2179 = xnode "Get Trap Data"("FPGA VI Reference In"=w3197, "error in"=w3196, "Number of Elements"=w3259, "Timeout (ms)"=-1 ("Timeout")) -> ("FPGA VI Reference Out"=w3092:T20, "error out"=w3091:errorcluster, "Data"=w3158:i16[], "Elements Remaining"=w3382:u32)
    "FIFO El. Rem." <- w3382
    n2180 = local read "DMA Update Period (s)"() -> (w3260:dbl)
    n2181 = local read "Trap AI FIFO Depth"() -> (w3384:u32)
    n2182 = local read "Number of APDs"() -> (w3060:u8)
    n2183 = Decimate 1D Array(w3157) -> (w3154:u16[], w3156:u16[], w3155:u16[])
    n2184 = feedback #3(0.0) -> (w3186:dbl)
    n2185 = Add(x=w3260, y=w3186) -> (x+y=w3358:dbl)
    n2186 = feedback-in #3(w3358) -> ()
    n2187 = To Time Stamp(1:w3186) -> (0:w3185:timestamp)
    n2188 = Subtract(x=w3384, y=w3259) -> (x-y=w3383:u32)
    n2189 = To Unsigned Long Integer(number=w3154) -> (unsigned 32bit integer=w3153:u32[])
    n2190 = Join Numbers(hi=w3156, lo=w3155) -> ((hi.lo)=w3152:u32[])
    n2191 = Divide(x=w3382, y=w3383) -> (x/y=w3381:dbl)
    "Buffer Status" <- w3381
    n2192 = case "Deinterlace APD signals" shown="3, Default" w3060 {
      tunnel: [w3394 w3400] -> w3037
      tunnel: w3228 -> [w3395 w3399]
      tunnel: [w3393 w3398] -> w3036
      tunnel: [w3392 w3396] -> w3043
      frame 3, Default {
        n2193 = Decimate 1D Array "APD signals"(w3395) -> (w3394:u32[], w3393:u32[], w3392:u32[])
      }
      frame 2 {
        n2194 = Decimate 1D Array "APD signals"(w3399) -> (w3400:u32[], w3398:u32[])
        n2195 = Multiply(x=w3398, y=u32 0) -> (x*y=w3396:u32[])
      }
    }
    n2196 = Join Numbers(hi=w3153, lo=w3152) -> ((hi.lo)=w3146:u64[])
    n2197 = call "IR AOM word to freq - vec.vi"("Frequency Word In (double vec)"=w3146) -> ("Frequency Out"=w3192:dbl[])
    n2198 = Equal?(x=w3381, y=1.0) -> (x = y?=w3379:bool)
    n2199 = case "Alert buffer overflow" shown="True" w3379 {
      frame False {
      }
      frame True {
        n2200 = call <vilib>:"Beep.vi"() -> ()  [unwired: 3 in, 9 out]
        "Overflow (data lost)" <- TRUE ("Overflow (data lost)")
      }
    }
    n2201 = Decimate 1D Array(w3192) -> (w3191:dbl[], w3190:dbl[])
    n2202 = Build Array(w3191, w3190) -> (w3189:dbl[][])
    n2203 = Bundle(w3037, w3036, w3043) -> (w3041:cluster{u32[], u32[], u32[]})  [unwired: 1 in]
    n2204 = Build Array(w3037, w3036, w3043) -> (w3318:u32[][])
    n2205 = for {
      tunnel: w3037 -> [w3390] mode=indexing
      n2206 = call "Smart Buffer (DBL) 1.vi"("new element [write]"=w3390, "mode"=T21."write") -> ()  [unwired: 4 in, 6 out]
    }
    n2207 = local read "APD Integration Time (s)"() -> (w3053:dbl)
    n2208 = To Double Precision Float(number=w3318) -> (double precision float=w3319:dbl[][])
    n2209 = feedback #4 "APD3"(w3043) -> (w3059:u32[])
    n2210 = feedback #5 "APD2"(w3036) -> (w3215:u32[])
    n2211 = feedback #6 "APD1"(w3037) -> (w3317:u32[])
    n2212 = Build Array (concatenate)(w3215, w3036) -> (w3214:u32[])
    n2213 = Build Array (concatenate)(w3059, w3043) -> (w3058:u32[])
    n2214 = Build Array (concatenate)(w3317, w3037) -> (w3314:u32[])
    n2215 = for {
      tunnel: w3036 -> [w3389] mode=indexing
      n2216 = call "Smart Buffer (DBL) 2.vi"("new element [write]"=w3389, "mode"=T21."write") -> ()  [unwired: 4 in, 6 out]
    }
    n2217 = Array Size(array=w3314) -> (size(s)=w3311:i32)
    n2218 = Array Size(array=w3037) -> (size(s)=w3313:i32)
    n2219 = Multiply(x=w3313, y="APD Ave N") -> (x*y=w3312:dbl)
    n2220 = Greater?(x=w3311, y=w3312) -> (0:w3315:bool)
    n2221 = Bundle("APD 1", "APD 2", "APD 3") -> (w3351:cluster{string, string, string})  [unwired: 1 out]
    n2222 = local read "Trap Sets"() -> (w3258:u32)
    n2223 = case shown="True" w3315 {
      tunnel: w3314 -> [w3698 w3707]
      tunnel: [w3698 w3705] -> w3265
      tunnel: w3312 -> [_ w3700]
      tunnel: w3311 -> [_ w3706]
      tunnel: w3214 -> [w3697 w3704]
      tunnel: [w3697 w3703] -> w3212
      tunnel: w3058 -> [w3696 w3702]
      tunnel: [w3696 w3699] -> w3054
      frame False {
      }
      frame True {
        n2224 = Subtract(x=w3706, y=w3700) -> (x-y=w3701:dbl)
        n2225 = Array Subset "APD3"(array=w3702, index=w3701, length=w3700) -> (w3699:u32[])
        n2226 = Array Subset "APD2"(array=w3704, index=w3701, length=w3700) -> (w3703:u32[])
        n2227 = Array Subset "APD1"(array=w3707, index=w3701, length=w3700) -> (w3705:u32[])
      }
    }
    n2228 = feedback-in #4(w3054) -> ()
    n2229 = feedback-in #5(w3212) -> ()
    n2230 = feedback-in #6(w3265) -> ()
    n2231 = Cluster To Array(cluster=w3351) -> (array=w3348:string[])
    n2232 = for "APD" {
      tunnel: w3319 -> [w3954] mode=indexing
      tunnel: w3053 -> [w3961]
      tunnel: [w3957] -> w3216 mode=indexing
      tunnel: "APD Disp. Scale" -> [w3958]
      tunnel: w3348 -> [w3956] mode=indexing
      tunnel: "APD Disp. Downsample" -> [w3952]
      tunnel: [w3955] -> w3347
      workers-P: _ -> [_]
      tunnel: w3185 -> [w3951]
      n2233 = call "integrate 1D array interval - double.vi"("Ave N"=w3952, "Array In"=w3954) -> ("Array Out"=w3953:dbl[])  [unwired: 1 out]
      n2234 = Multiply(x=w3961, y=w3952) -> (x*y=w3955:dbl)
      n2235 = Divide(x=w3953, y=w3958) -> (x/y=w3959:dbl[])
      n2236 = Bundle By Name("t0"=w3951, "Y"=w3959, "dt"=w3955) -> (w3960:waveform(dbl))  [unwired: 1 out]
      n2237 = Set Waveform Attribute(5:w3956, 6:"NI_ChannelName" ("name"), 7:w3960) -> (3:w3957:waveform(dbl))  [unwired: 1 in, 2 out]
    }
    "APD Display Period (s)" <- w3347
    n2238 = Reciprocal(x=w3347) -> (1/x=→"APD Display Freq. (Hz)":dbl)
    n2239 = case "Deinterlace trap data, average down PSD" shown="2" w3258 {
      tunnel: w3158 -> [w3979 w4044]
      tunnel: [w3976 w4041] -> w3251
      tunnel: [w3979 w4043] -> w3149
      tunnel: "Detector Type" -> [w3978 w4039]
      tunnel: [w3977 w4042] -> w3250
      tunnel: [w3975 w4040] -> w3356
      frame 1, Default {
        n2240 = Divide(x=w3979, y=3276.7) -> (x/y=w3980:dbl[])
        n2241 = Decimate 1D Array(w3980) -> (w3989:dbl[], w3988:dbl[], w3987:dbl[], w3986:dbl[], w3985:dbl[], w3984:dbl[], w3983:dbl[], w3982:dbl[])
        n2242 = case shown="\"IR-QPD + PSD + FB-QPD position\"" w3978 {
          tunnel: w3989 -> [w4013 w4038]
          tunnel: w3988 -> [w4012 w4037]
          tunnel: w3987 -> [w3997 w4015]
          tunnel: w3986 -> [w3998 w4025]
          tunnel: w3985 -> [w4011 w4036]
          tunnel: w3984 -> [w4010 w4035]
          tunnel: w3983 -> [w3994 w4016]
          tunnel: w3982 -> [w3993 w4014]
          tunnel: [w3992 w4022] -> w3977
          tunnel: [w3991 w4021] -> w3976
          tunnel: [w3990 w4020] -> w3975
          frame "IR-QPD + PSD + FB-QPD", Default {
            w3990 = 0  # Channel pattern
            n2243 = Divide(x=w4013, y=w3998) -> (x/y=w4000:dbl[])
            n2244 = Divide(x=w4012, y=w3998) -> (x/y=w3999:dbl[])
            n2245 = Divide(x=w4011, y=w3994) -> (x/y=w3996:dbl[])
            n2246 = Divide(x=w4010, y=w3993) -> (x/y=w3995:dbl[])
            n2247 = Build Array(w4000, w3999, w3998, w3997, w3996, w3995, w3994, w3993) -> (w3991:dbl[][])
            n2248 = Bundle("T1 Y", "T1 X", "T1 Sum", "FB Sum", "PSD Y", "PSD X", "PSD Y Sum", "PSD X Sum") -> (w4009:T40)  [unwired: 1 out]
            n2249 = Cluster To Array(cluster=w4009) -> (array=w3992:string[])
          }
          frame "IR-QPD + PSD + FB-QPD position" {
            w4020 = 3  # Channel pattern
            n2250 = Negate(x=w4016) -> (-x=w4017:dbl[])
            n2251 = Divide(x=w4038, y=w4025) -> (x/y=w4027:dbl[])
            n2252 = Divide(x=w4037, y=w4025) -> (x/y=w4026:dbl[])
            n2253 = Divide(x=w4036, y=w4016) -> (x/y=w4024:dbl[])
            n2254 = Divide(x=w4035, y=w4017) -> (x/y=w4023:dbl[])
            n2255 = Build Array(w4027, w4026, w4025, w4014, w4015, w4024, w4023, w4016) -> (w4021:dbl[][])
            n2256 = Bundle("T1 Y", "T1 X", "T1 Sum", "FB X", "FB Sum", "PSD Y", "PSD X", "PSD Y Sum") -> (w4034:T40)  [unwired: 1 out]
            n2257 = Cluster To Array(cluster=w4034) -> (array=w4022:string[])
          }
        }
      }
      frame 2 {
        n2258 = case shown="\"IR-QPD + PSD + FB-QPD X position\"" w4039 {
          tunnel: w4044 -> [w4106 w4178 w4249]
          tunnel: [w4045 w4169 w4180] -> w4043
          tunnel: [w4072 w4160 w4227] -> w4042
          tunnel: [w4071 w4123 w4194] -> w4041
          tunnel: [w4065 w4158 w4225] -> w4040
          frame "IR-QPD + PSD + FB-QPD", Default {
            w4065 = 1  # Channel pattern
            # "time average x2 the 4th signal and the 4 psd signals (detection laser)"
            # "deinterlace 3 signals from qpd"
            n2259 = Decimate 1D Array(w4106) -> (w4105:i16[], w4104:i16[], w4070:i16[], w4103:i16[], w4093:i16[], w4091:i16[], w4090:i16[], w4088:i16[])
            n2260 = Decimate 1D Array(w4070) -> (w4069:i16[], w4068:i16[])
            n2261 = Decimate 1D Array(w4105) -> (w4102:i16[], w4074:i16[])
            n2262 = Decimate 1D Array(w4104) -> (w4101:i16[], w4099:i16[])
            n2263 = Decimate 1D Array(w4103) -> (w4100:i16[], w4098:i16[])
            n2264 = call "downsample 1D array - double.vi"("Ave N"=2.0, "Array In"=w4093) -> ("Array Out"=w4092:dbl[])  [unwired: 1 out]
            n2265 = call "downsample 1D array - double.vi"("Ave N"=2.0, "Array In"=w4091) -> ("Array Out"=w4073:dbl[])  [unwired: 1 out]
            n2266 = call "downsample 1D array - double.vi"("Ave N"=2.0, "Array In"=w4090) -> ("Array Out"=w4089:dbl[])  [unwired: 1 out]
            n2267 = call "downsample 1D array - double.vi"("Ave N"=2.0, "Array In"=w4088) -> ("Array Out"=w4087:dbl[])  [unwired: 1 out]
            n2268 = Interleave 1D Arrays(w4102, w4101, w4100, w4074, w4099, w4098, w4069, w4068, w4092, w4073, w4089, w4087) -> (w4086:dbl[])
            n2269 = Divide(x=w4086, y=3276.7) -> (x/y=w4085:dbl[])
            n2270 = Decimate 1D Array(w4085) -> (w4084:dbl[], w4083:dbl[], w4082:dbl[], w4081:dbl[], w4080:dbl[], w4079:dbl[], w4067:dbl[], w4066:dbl[], w4078:dbl[], w4077:dbl[], w4076:dbl[], w4075:dbl[])
            n2271 = Divide(x=w4084, y=w4082) -> (x/y=w4052:dbl[])
            n2272 = Divide(x=w4083, y=w4082) -> (x/y=w4051:dbl[])
            n2273 = Divide(x=w4081, y=w4079) -> (x/y=w4050:dbl[])
            n2274 = Divide(x=w4080, y=w4079) -> (x/y=w4049:dbl[])
            n2275 = Divide(x=w4078, y=w4076) -> (x/y=w4048:dbl[])
            n2276 = Divide(x=w4077, y=w4075) -> (x/y=w4047:dbl[])
            n2277 = Build Array(w4052, w4051, w4082, w4050, w4049, w4079, w4067, w4066, w4048, w4047, w4076, w4075) -> (w4071:dbl[][])
            n2278 = Bundle("T1 Y", "T1 X", "T1 Sum", "T2 Y", "T2 X", "T2 Sum", "T1 FB Sum", "T2 FB Sum", "PSD Y", "PSD X", "PSD Y Sum", "PSD X Sum") -> (w4053:T41)  [unwired: 1 out]
            n2279 = To Word Integer(number=w4086) -> (16bit integer=w4045:i16[])
            n2280 = Cluster To Array(cluster=w4053) -> (array=w4072:string[])
          }
          frame "IR-QPD + PSD + FB-QPD X position" {
            w4158 = 2  # Channel pattern
            # "time average x2 the 3 psd signals (detection laser)"
            # "deinterlace 3 signals from qpds"
            n2281 = Decimate 1D Array(w4178) -> (w4177:i16[], w4176:i16[], w4159:i16[], w4175:i16[], w4121:i16[], w4118:i16[], w4115:i16[], w4146:i16[])
            n2282 = Select(t=i16 -1, s="Flip X Sign", f=i16 1) -> (s? t:f=w4111:i16)
            n2283 = Multiply(x=w4176, y=w4111) -> (x*y=w4112:i16[])
            n2284 = Decimate 1D Array(w4159) -> (w4144:i16[], w4142:i16[])
            n2285 = Decimate 1D Array(w4177) -> (w4174:i16[], w4161:i16[])
            n2286 = Decimate 1D Array(w4112) -> (w4173:i16[], w4171:i16[])
            n2287 = Decimate 1D Array(w4175) -> (w4172:i16[], w4170:i16[])
            n2288 = Decimate 1D Array(w4146) -> (w4145:i16[], w4143:i16[])
            n2289 = call "downsample 1D array - I16.vi"("Ave N"=2.0, "Array In"=w4121) -> ("Array Out"=w4119:i16[])  [unwired: 1 in]
            n2290 = call "downsample 1D array - I16.vi"("Ave N"=2.0, "Array In"=w4115) -> ("Array Out"=w4113:i16[])  [unwired: 1 in]
            n2291 = call "downsample 1D array - I16.vi"("Ave N"=2.0, "Array In"=w4118) -> ("Array Out"=w4116:i16[])  [unwired: 1 in]
            n2292 = Interleave 1D Arrays(w4174, w4173, w4172, w4161, w4171, w4170, w4145, w4144, w4143, w4142, w4119, w4116, w4113) -> (w4169:i16[])
            n2293 = Divide(x=w4169, y=3276.7) -> (x/y=w4168:dbl[])
            n2294 = Decimate 1D Array(w4168) -> (w4167:dbl[], w4166:dbl[], w4165:dbl[], w4164:dbl[], w4163:dbl[], w4162:dbl[], w4134:dbl[], w4132:dbl[], w4131:dbl[], w4129:dbl[], w4128:dbl[], w4127:dbl[], w4124:dbl[])
            n2295 = Negate(x=w4124) -> (-x=w4122:dbl[])
            n2296 = Divide(x=w4128, y=w4124) -> (x/y=w4126:dbl[])
            n2297 = Divide(x=w4127, y=w4122) -> (x/y=w4125:dbl[])
            n2298 = Divide(x=w4167, y=w4165) -> (x/y=w4150:dbl[])
            n2299 = Divide(x=w4166, y=w4165) -> (x/y=w4149:dbl[])
            n2300 = Divide(x=w4164, y=w4162) -> (x/y=w4148:dbl[])
            n2301 = Divide(x=w4163, y=w4162) -> (x/y=w4147:dbl[])
            n2302 = Divide(x=w4134, y=w4132) -> (x/y=w4133:dbl[])
            n2303 = Divide(x=w4131, y=w4129) -> (x/y=w4130:dbl[])
            n2304 = Build Array(w4150, w4149, w4165, w4148, w4147, w4162, w4133, w4132, w4130, w4129, w4126, w4125, w4124) -> (w4123:dbl[][])
